vi "HandleRollerMotor.vi"(8 "error in":errorcluster, 9 "JoystickValue":dbl) -> (0 "error out":errorcluster, 2 "StateOut":T1)   [LabVIEW 2013]
doc: "If Joystick Values is not equal to 0 then if it is > 0 do Forward State. if < 0 then ReverseState.\nOtherwiae go to OffState"
uses:
  RollerAction.ctl
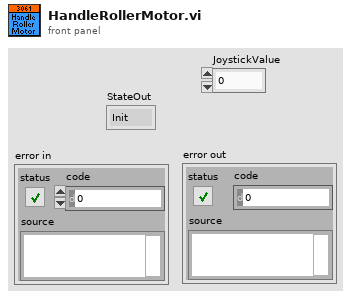
[diagram p1: front panel]
types:
  T1 = typedef "RollerAction.ctl" = enum16{"Init", "Off", "Forward", "Reverse"}
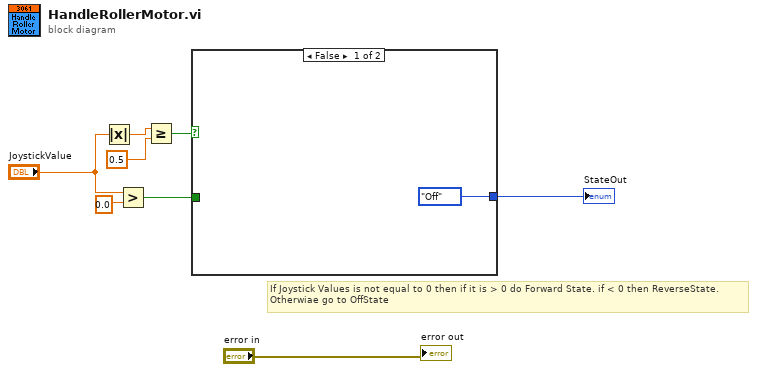
[diagram p0: block diagram]
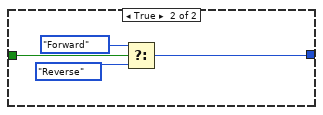
[diagram p2: hidden frame]
diagram:
  # "If Joystick Values is not equal to 0 then if it is > 0 do Forward State. if < 0 then ReverseState.\nOtherwiae go to OffState"
  n1 = Absolute Value(x="JoystickValue") -> (abs(x)=w3:dbl)
  n2 = Greater?(x="JoystickValue", y=0.0) -> (0:w6:bool)
  n3 = Greater Or Equal?(x=w3, y=0.5) -> (x >= y?=w1:bool)
  n4 = case shown="False" w1 {
    tunnel: [RollerAction."Off" ("OffState") w13] -> w5
    tunnel: w6 -> [_ w12]
    frame False {
    }
    frame True {
      n5 = Select(t=RollerAction."Forward" ("ForwardState"), s=w12, f=RollerAction."Reverse" ("ReverseState")) -> (s? t:f=w13:T1)
    }
  }
  "StateOut" <- w5
  "error out" <- "error in"
